vi "Project2.vi"() -> ()   [LabVIEW 2024]
panel:
  out "Pump":bool
  out "System":bool
  out "Height (cm)":dbl(slide) scale=0.0..60.0
  out "Low Pressure":bool
  in  "stop":bool
  out "Pressure in H2O":dbl(slide) scale=0.0..25.0
  out "Amps, mA":dbl(slide) scale=0.0..25.0
  out "AtoD Hex":i16 format="%x"
  out "AtoD":dbl
  out "SCC,V":dbl(slide) scale=0.0..7.0
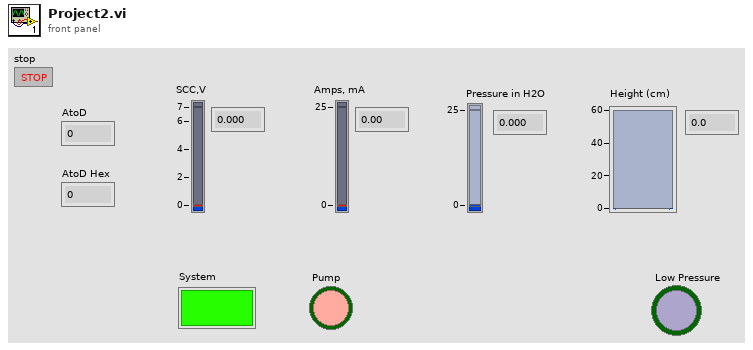
[diagram p1: front panel]
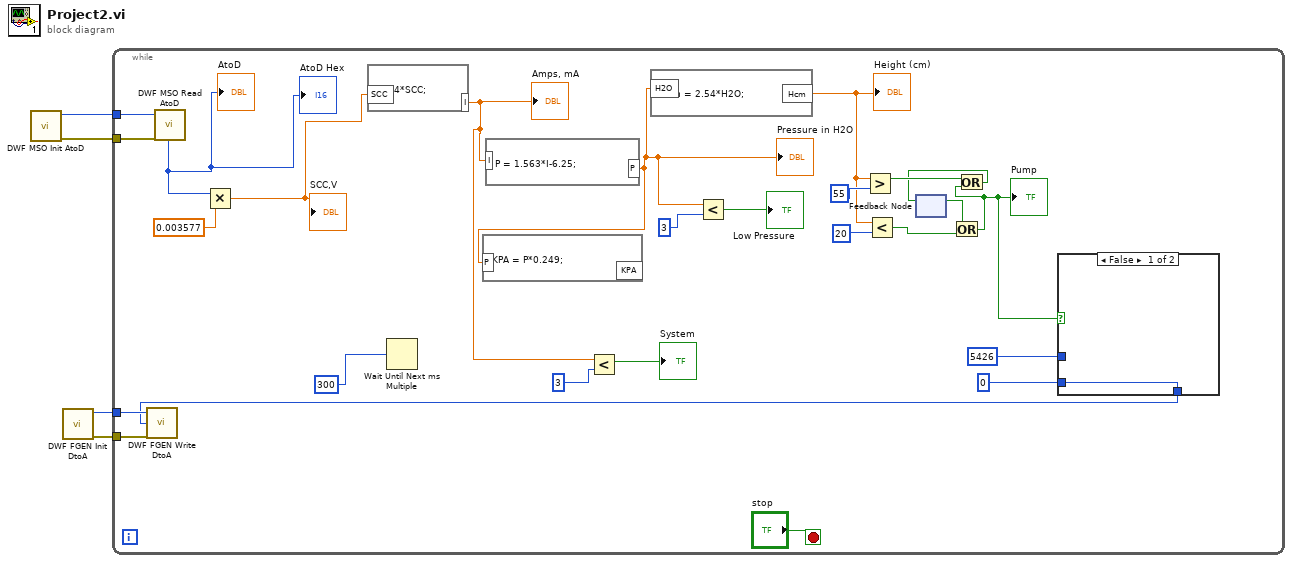
[diagram p0: block diagram]
diagram:
  n1 = call "DWF MSO Init AtoD.vi"() -> ("Error Out"=w3:errorcluster, "Instrument Handle Out"=w4:u32)  [unwired: 10 in]
  n2 = call "DWF FGEN Init DtoA.vi"() -> ("Error Out"=w1:errorcluster, "Instrument Handle Out"=w2:u32)  [unwired: 10 in]
  n3 = while {
    tunnel: w4 -> [w30]
    tunnel: w3 -> [w29]
    tunnel: w2 -> [w10]
    tunnel: w1 -> [w9]
    stop <- "stop" stop-if-true
    n4 = call "DWF MSO Read AtoD.vi"("Instrument Handle In AtoD"=w30, "Error In"=w29) -> ("AtoD"=w27:i16)  [unwired: 12 in, 1 out]
    "AtoD" <- w27
    "AtoD Hex" <- w27
    n5 = Multiply(x=w27, y=0.003577) -> (x*y=w26:dbl)
    "SCC,V" <- w26
    n6 = formula code="I = 4*SCC;"("SCC"=w26) -> ("I"=w21:dbl)
    "Amps, mA" <- w21
    n7 = Wait Until Next ms Multiple(millisecond multiple=300) -> ()  [unwired: 1 out]
    n8 = formula code="P = 1.563*I-6.25;"("I"=w21) -> ("P"=w5:dbl)
    "Pressure in H2O" <- w5
    n9 = formula code="KPA = P*0.249;"("P"=w5) -> ()  [unwired: 1 out]
    n10 = Less?(x=w21, y=3) -> (x < y?=→"System":bool)
    n11 = formula code="Hcm = 2.54*H2O;"("H2O"=w5) -> ("Hcm"=w15:dbl)
    "Height (cm)" <- w15
    n12 = Less?(x=w5, y=3) -> (x < y?=→"Low Pressure":bool)
    n13 = Greater?(x=w15, y=55) -> (0:w19:bool)
    n14 = Less?(x=w15, y=20) -> (x < y?=w18:bool)
    n15 = feedback #1() -> (w13:bool)  [unwired: 1 in]
    n16 = Or(x=w13, y=w18) -> (x .or. y?=w11:bool)
    "Pump" <- w11
    n17 = Or(x=w19, y=w11) -> (x .or. y?=w14:bool)
    n18 = feedback-in #1(w14) -> ()
    n19 = case shown="False" w11 {
      tunnel: 5426 -> [_ w32]
      tunnel: [w31 w32] -> w6
      tunnel: 0 -> [w31 _]
      frame False {
      }
      frame True {
      }
    }
    n20 = call "DWF FGEN Write DtoA.vi"("Error In"=w9, "Raw Data"=w6, "Instrument Handle In"=w10) -> ()  [unwired: 1 in, 2 out]
  }
